vi "UI Test.vi"() -> ()   [LabVIEW 2014]
uses:
  Reusable/CRDS/Data/Main/CRDS Data.lvclass
  Reusable/CRDS/Data/Main/Read CellData.vi
  Reusable/CRDS/Data/Cell/Read Ringdowns.vi
  Reusable/CRDS/Data/Cell/CRDS Cell Data.lvclass
panel:
  out "Waveform Graph":i16[][](graph)
  in  "index (page)":i32
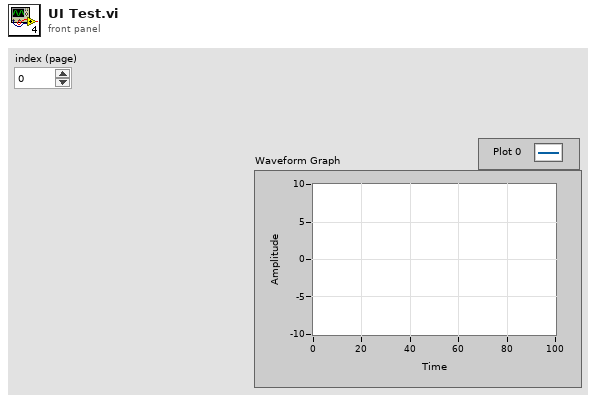
[diagram p1: front panel]
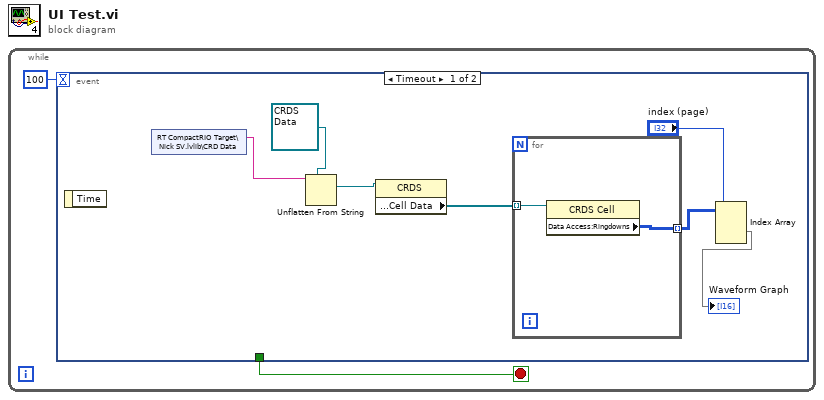
[diagram p0: block diagram]
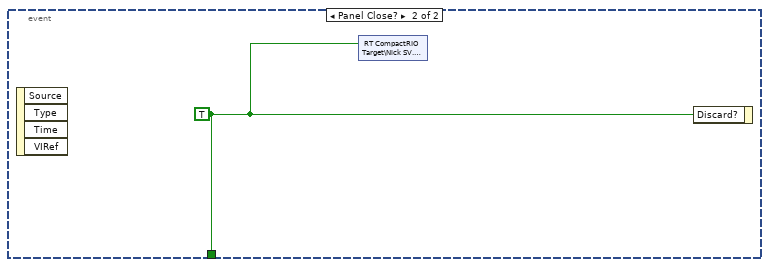
[diagram p2: hidden frame]
diagram:
  n1 = while {
    stop <- w1 stop-if-true
    n2 = event shown="[0] Timeout" {
      selector: _ -> [_ _]
      dyn-events: _ -> [_ _]
      timeout: 100 -> [_ _]
      tunnel: [_ w12] -> w1
      event Timeout {
        n3 = event-data() -> ()  [unwired: 1 in, 1 out]
        n4 = shared-variable "RT CompactRIO Target\\Nick SV.lvlib\\CRD Data"() -> (w9:string)  [unwired: 1 in, 1 out]
        n5 = Unflatten From String(type=refnum<class "CRDS Data.lvclass"> refnum ("CRDS"), binary string=w9) -> (value=w7:refnum<class "CRDS Data.lvclass">)  [unwired: 3 in, 2 out]
        n6 = property class="CRDS"(reference=w7) -> ("Data Access:Cell Data"=w6:refnum<class "CRDS Cell Data.lvclass">[])  [unwired: 1 in, 2 out]
        n7 = for {
          tunnel: w6 -> [w11] mode=indexing
          tunnel: [w10] -> w5 mode=indexing
          n8 = property class="CRDS Cell"(reference=w11) -> ("Data Access:Ringdowns"=w10:i16[][])  [unwired: 1 in, 2 out]
        }
        n9 = Index Array(array=w5, index (dim 0)="index (page)") -> (element=→"Waveform Graph":i16[][])  [unwired: 2 in]
      }
      event Panel Close? {
        w12 = TRUE ("Discard?")
        n10 = event-data() -> ()  [unwired: 1 in, 4 out]
        n11 = shared-variable "RT CompactRIO Target\\Nick SV.lvlib\\Stop"(w12) -> ()  [unwired: 1 in, 1 out]
        n12 = event-data("Discard?"=w12) -> ()  [unwired: 1 in, 1 out]
      }
    }
  }
